vi "CoMP-S Objective Lens Calculate.vi"(5 "file path (use dialog)":path=path "C:/CoMP-S Observer/focus.txt", 7 "error in (no error)":errorcluster, 9 "old Focus":T1=70.0 min=15.0 max=155.0 format="%.2f", 10 "new Focus":T1=70.0 min=15.0 max=155.0 format="%.2f") -> (0 "error out":errorcluster, 1 "Velocity":i32, 2 "Motor Direction":bool=TRUE, 3 "Steps":i32)   [LabVIEW 2014]
doc: "VI for computig velocity and direction of focus motor moving. \n\nThe program is loading value from file and compare with new value,while velocity and motor direction are output indicators. Finally is old value in file replaced by new one."
uses:
  Controls/focus.ctl
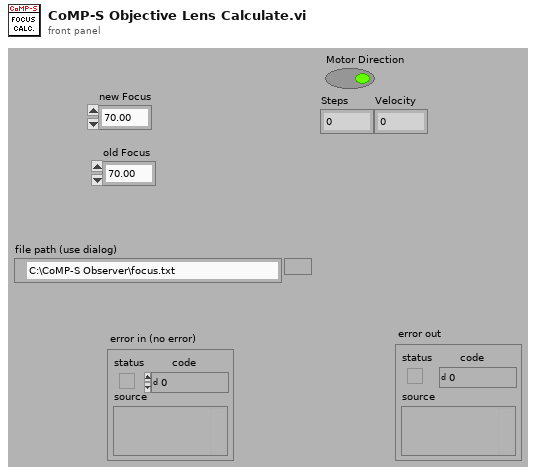
[diagram p1: front panel]
types:
  T1 = typedef "focus.ctl" = dbl
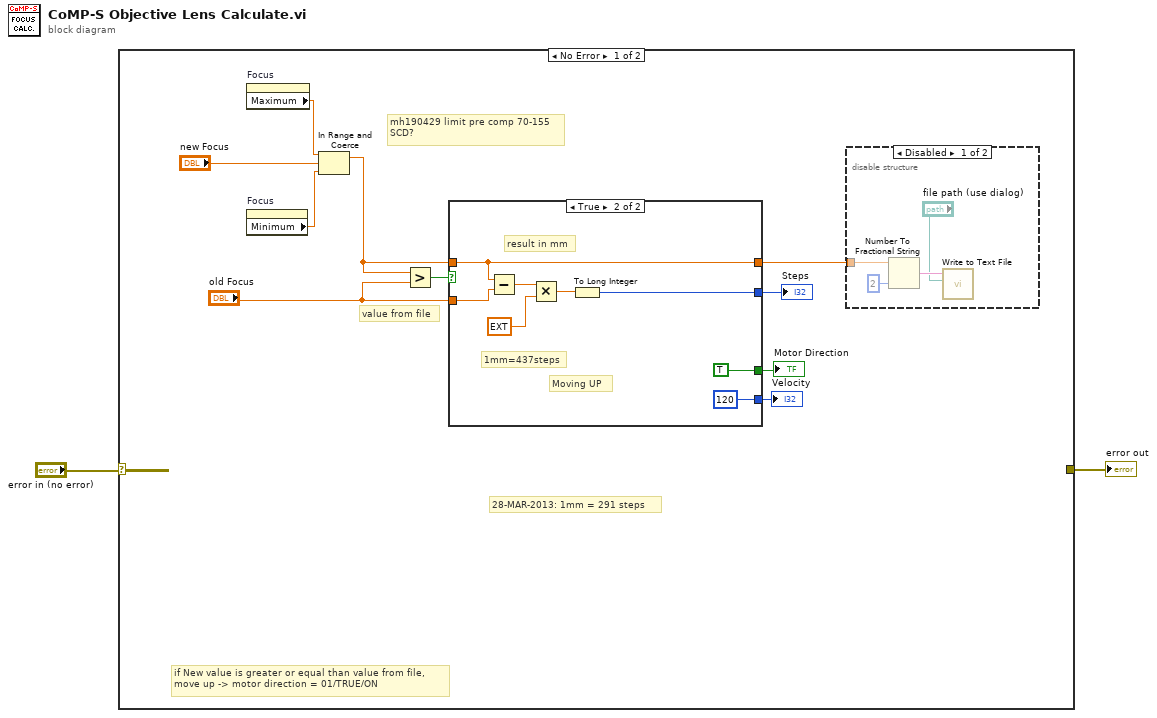
[diagram p0: block diagram]
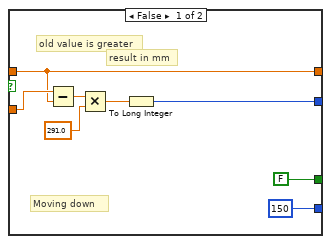
[diagram p3: hidden frame]
diagram:
  n1 = case shown="No Error" "error in (no error)" {
    selector: "error in (no error)" -> [_ w33]
    tunnel: [_ w33] -> w1
    frame No Error {
      # "mh190429 limit pre comp 70-155\nSCD?"
      # "28-MAR-2013: 1mm = 291 steps"
      # "if New value is greater or equal than value from file, \nmove up -> motor direction = 01/TRUE/ON"
      # "value from file"
      n2 = property on="Focus" class="DigNum (strict)"() -> ("Maximum"=w5:dbl)  [unwired: 2 in, 2 out]
      n3 = property on="Focus" class="DigNum (strict)"() -> ("Minimum"=w4:dbl)  [unwired: 2 in, 2 out]
      n4 = In Range and Coerce(upper limit=w5, x="new Focus", lower limit=w4) -> (coerced(x)=w7:T1)  [unwired: 1 out]
      n5 = Greater?(x=w7, y="old Focus") -> (0:w10:bool)
      n6 = case shown="True" w10 {
        tunnel: w7 -> [w18 w26]
        tunnel: "old Focus" -> [w24 w32]
        tunnel: [FALSE TRUE] -> w11
        tunnel: [w20 w27] -> w12
        tunnel: [w18 w26] -> w9
        tunnel: [150 120] -> w8
        frame False {
          # "Moving down"
          # "result in mm"
          # "old value is greater"
          n7 = Subtract(x=w24, y=w18) -> (x-y=w23:T1)
          n8 = Multiply(x=w23, y=291.0) -> (x*y=w21:T1)
          n9 = To Long Integer(number=w21) -> (32bit integer=w20:i32)
        }
        frame True {
          # "Moving UP"
          # "1mm=437steps"
          # "result in mm"
          n10 = Subtract(x=w26, y=w32) -> (x-y=w31:T1)
          n11 = Multiply(x=w31, y=ext 291.0) -> (x*y=w29:ext)
          n12 = To Long Integer(number=w29) -> (32bit integer=w27:i32)
        }
      }
      "Motor Direction" <- w11
      "Steps" <- w12
      "Velocity" <- w8
      n13 = disable-structure shown="Disabled" {
        disable-tunnel: w9 -> [w14 _]
        frame Disabled {
          n14 = Number To Fractional String(number=w14, precision (6)=i16 2) -> (F-format string=w16:string)  [unwired: 2 in]
          n15 = call "Write to Text File.vi"("file path (use dialog)"="file path (use dialog)", "text"=w16) -> ()  [unwired: 9 in, 1 out]
        }
        frame Enabled {
        }
      }
    }
    frame Error {
    }
  }
  "error out" <- w1
